vi "Property Strings.vi"() -> ()   [LabVIEW 2015, in "Waveform Data Logger Shared.lvlib"]
uses:
  Waveform Data Logger Shared.lvlib
panel:
  in  "Minimum Buffer Size":string="Minimum Buffer Size"
  in  "Use Custom Buffer Size":string="Use Custom Buffer Size "
  in  "Multi Trigs":string="Multi Trigs"
  in  "Q size":string="Q size"
  in  "Auto Q size":string="Auto Q size"
  in  "Retriggerable":string="Retriggerable"
  in  "File Conflict Operation":string="File Conflict Operation"
  in  "Stop Trigger Channel":string="Stop Trigger Channel"
  in  "Start Trigger Channel":string="Start Trigger Channel"
  in  "Stop Default State":string="Stop Default State"
  in  "Start Default State":string="Start Default State"
  in  "Stop Digital Edge":string="Stop Digital Edge"
  in  "Start Digital Edge":string="Start Digital Edge"
  in  "Stop Analog Threshold":string="Stop Analog Threshold"
  in  "Stop Analog Slope":string="Stop Analog Slope"
  in  "Stop Analog Strict Edge":string="Stop Analog Strict Edge"
  in  "Start Analog Threshold":string="Start Analog Threshold"
  in  "Start Analog Slope":string="Start Analog Slope"
  in  "Start Analog Strict Edge":string="Start Analog Strict Edge"
  in  "Stop In Range Invert?":string="Stop  In Range Invert?"
  in  "Stop In Range Low Limit":string="Stop  In Range Low Limit"
  in  "Stop In Range High Limit":string="Stop In Range High Limit"
  in  "Start In Range Invert?":string="Start In Range Invert?"
  in  "Start In Range Low Limit":string="Start In Range Low Limit"
  in  "Start In Range High Limit":string="Start In Range High Limit"
  in  "Stop Value Change Deadband":string="Stop Value Change Deadband"
  in  "Start Value Change Deadband":string="Start Value Change Deadband"
  in  "Stop Boolean Operand":string="Stop Boolean Operand"
  in  "Stop Boolean Value":string="Stop Boolean Value"
  in  "Start Boolean Operand":string="Start Boolean Operand"
  in  "Start Boolean Value":string="Start Boolean Value"
  in  "Posttrigger Time":string="Posttrigger Time"
  in  "Ignore timestamps?":string="Ignore timestamps?"
  in  "Log Timeout":string="Log Timeout"
  in  "Use Log Name As Group":string="Use Log Name As Group"
  in  "Stop Trig":string="Stop Trig"
  in  "Start Trig":string="Start Trig"
  in  "Group Name":string="Group Name"
  in  "File Size Units":string="File Size Units"
  in  "File Size":string="Max File Size"
  in  "Span Multiple Files":string="Span Multiple Files"
  in  "Decimations":string="Decimations"
  in  "Log Wfm Names":string="Log Wfm Names"
  in  "Log Wfm Base":string="Log Wfm"
  in  "Pretrigger Time":string="Pretrigger Time"
  in  "Log File Path":string="Log File Path"
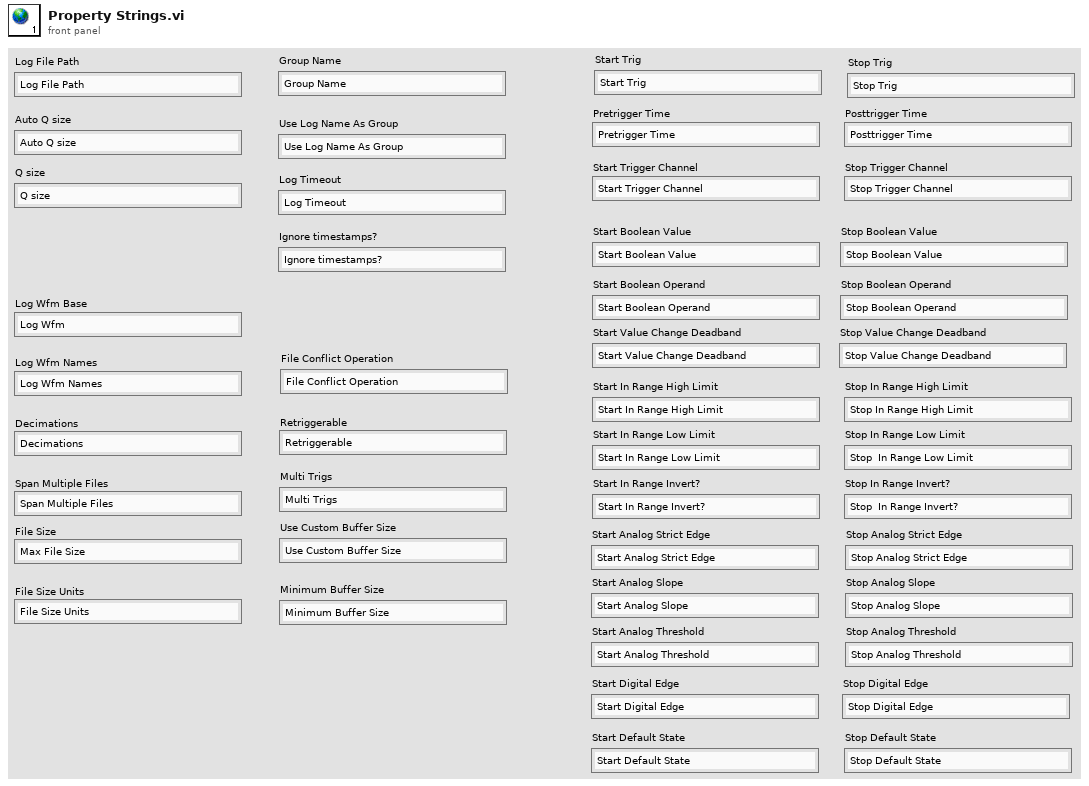
[diagram p1: front panel]
diagram:
